vi "Size_to_ROI.vi"(11 "Image Size":cluster{"X":i32, "Y":i32}) -> (3 "Rectangle":T1 {"Rotation" format="%.2f"; "Left" scale=0.0..1024.0; "Right" scale=0.0..1024.0})   [LabVIEW 2019]
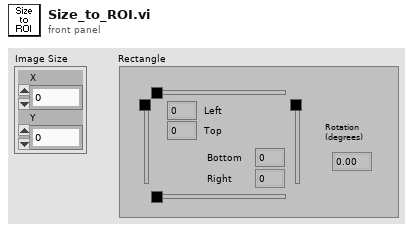
[diagram p1: front panel]
types:
  T1 = typedef "IMAQ Rectangle" = cluster{"Left":i32, "Top":i32, "Right":i32, "Bottom":i32, "Rotation":dbl}
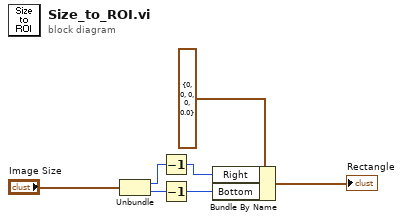
[diagram p0: block diagram]
diagram:
  n1 = Unbundle("Image Size") -> ("X"=w4:i32, "Y"=w5:i32)
  n2 = Decrement(x=w4) -> (x-1=w6:i32)
  n3 = Decrement(x=w5) -> (x-1=w7:i32)
  n4 = Bundle By Name(cluster=T1 {"Left"=0, "Top"=0, "Right"=0, "Bottom"=0, "Rotation"=0.0} ("Rectangle"), "Right"=w6, "Bottom"=w7) -> (→"Rectangle":T1)
